vi "CFTS (TDT).vi"() -> ()   [LabVIEW 2020]
uses:
  Human Studies/NSDH Frontend/LV Source/Typedefs/NSDH-Options.ctl
  CFTS Main Panel SubVIs/CFTS-Experiment State.ctl
  <vilib>/Utility/sysdir.llb/System Directory Type.ctl
  DPOAE VIs/DP Analysis Panel.vi
  DPOAE VIs/DP I-O Main Panel.vi
  Calibration VIs/Calibrate Probe Tube.vi
panel:
  in  "Options":bool
  in  "CalMenu":u16(ring) items=["Calibration", "In-ear", "Probe tube", "Headphone"]
  out "exit signal":bool
  in  "DevicesButton":bool
  in  "DPAnalysisButton":bool
  in  "DPButton":bool
  in  "Cancel Button":bool
  in  "ApplyButton":bool
  in  "ID":string
  in  "Number":i32
  in  "EphysBrowserButton":bool
  in  "EphysButton":bool
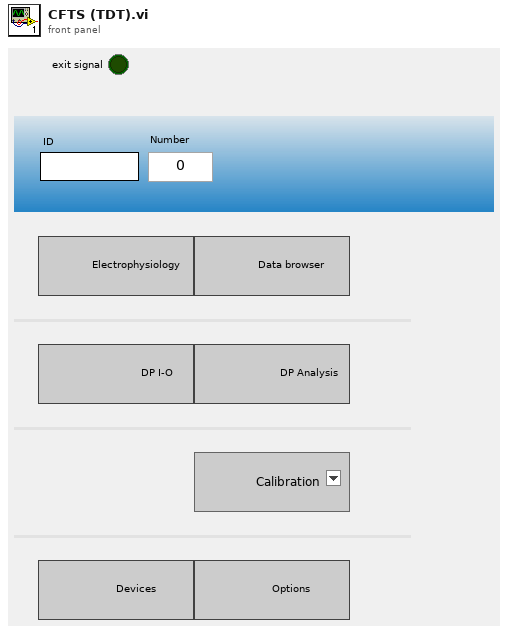
[diagram p1: front panel]
types:
  T1 = enum8{"Enabled", "Disabled", "Disabled and Grayed Out"}
  T2 = typedef "CFTS-Experiment State.ctl" = cluster{"Experimenter":string, "Number":u32, "Right":string, "Left":string, "Data Folder":path, "State File":path, "Version Info":string, "End Exposure Time":dbl, "Exposure Duration":string, "Run #":cluster{"CAP":i16, "ABR":i16, "DP":i16, "VsEP":i16, "MeasSeq":i16, "SubSeq":i16, "SFOAE":i16}}
  T3 = typedef "NSDH-Options.ctl" = cluster{"Data root":path}
  T4 = typedef "System Directory Type.ctl" = i32
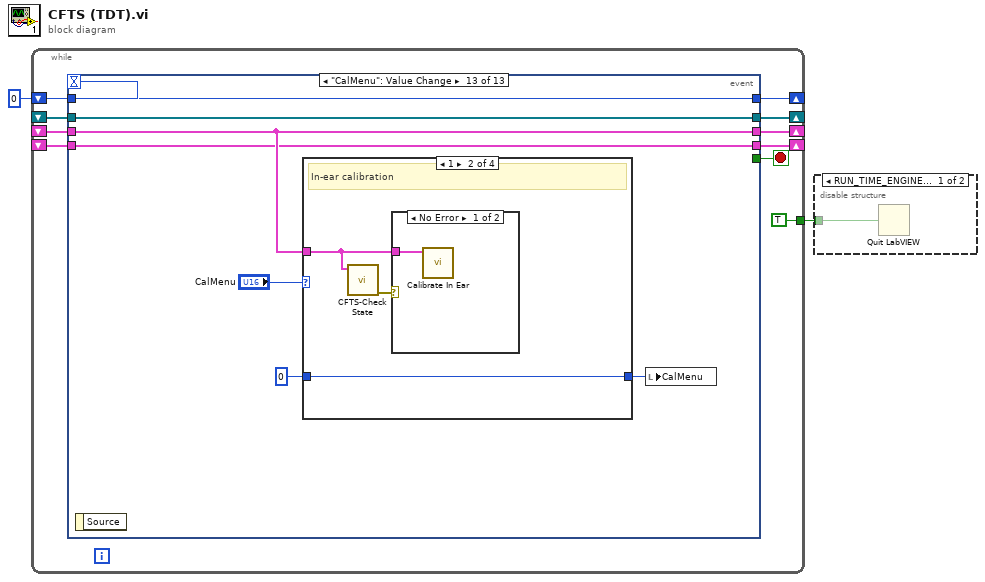
[diagram p0: block diagram]
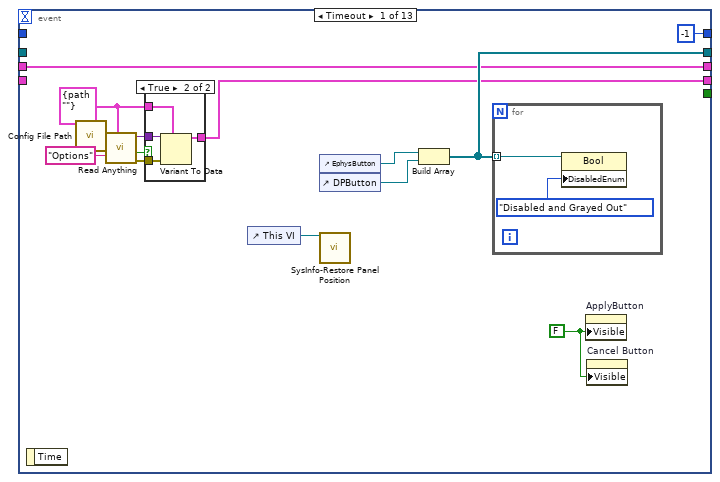
[diagram p3: hidden frame]
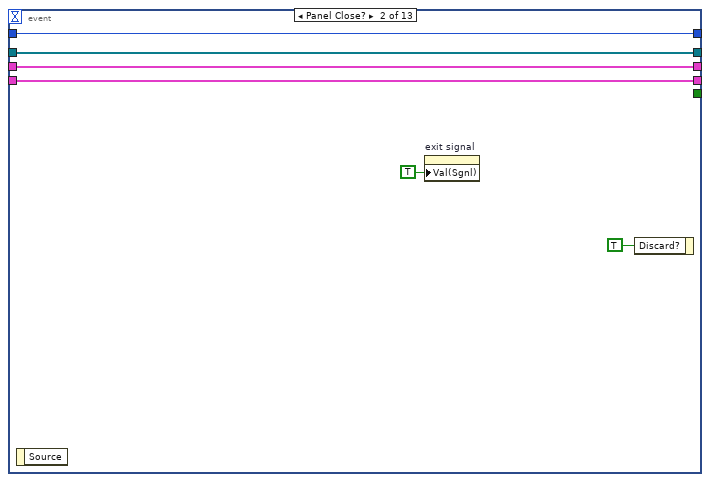
[diagram p5: hidden frame]
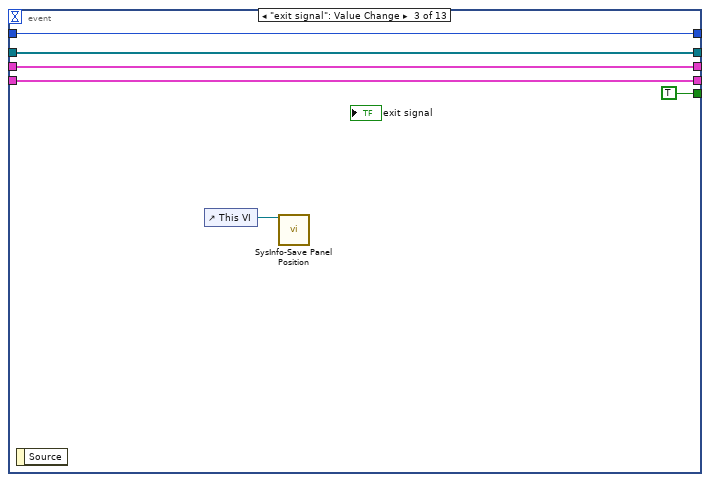
[diagram p6: hidden frame]
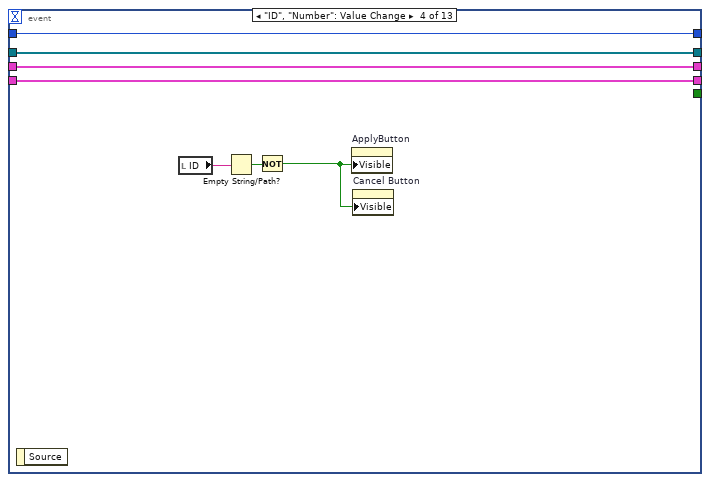
[diagram p7: hidden frame]
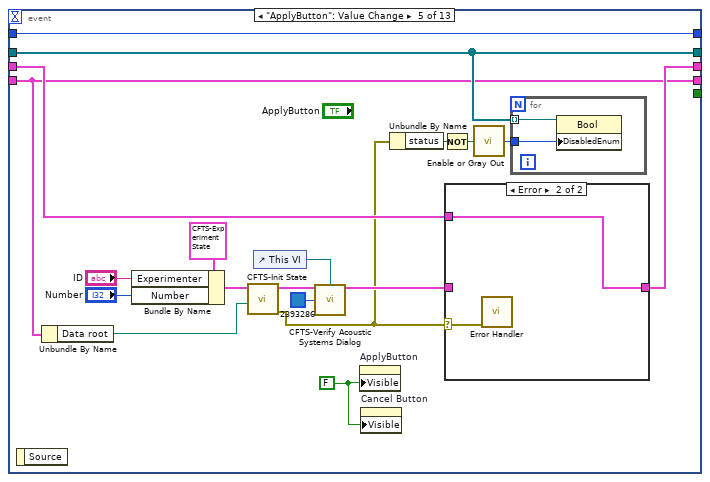
[diagram p8: hidden frame]
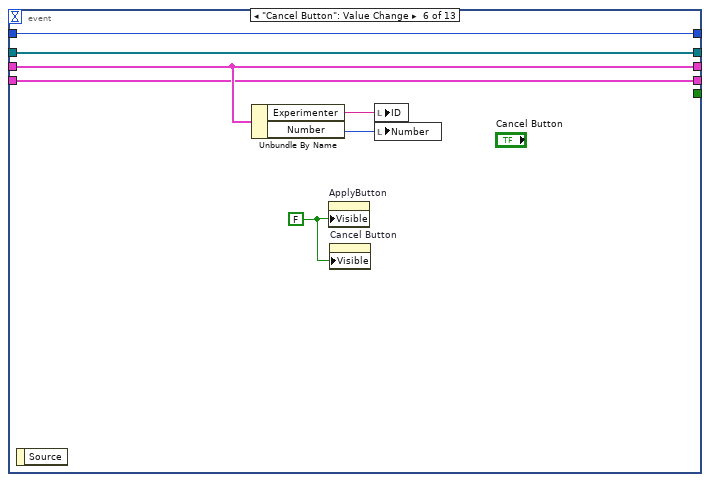
[diagram p10: hidden frame]
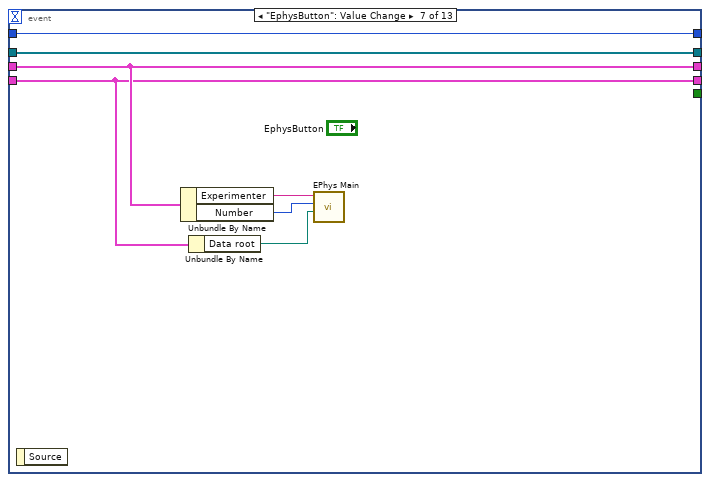
[diagram p11: hidden frame]
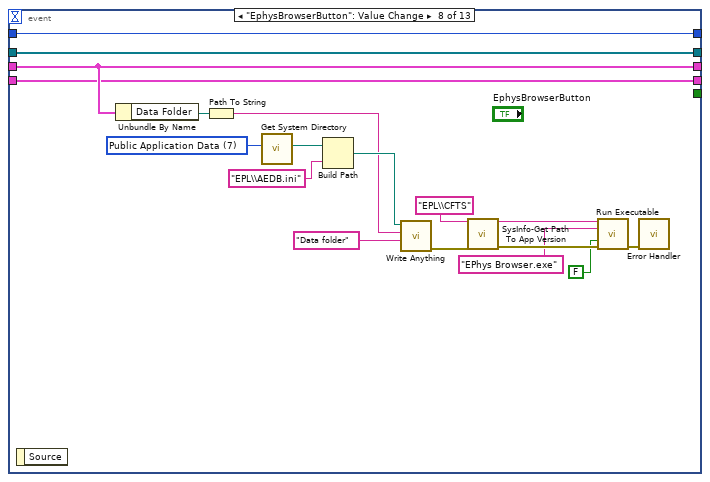
[diagram p12: hidden frame]
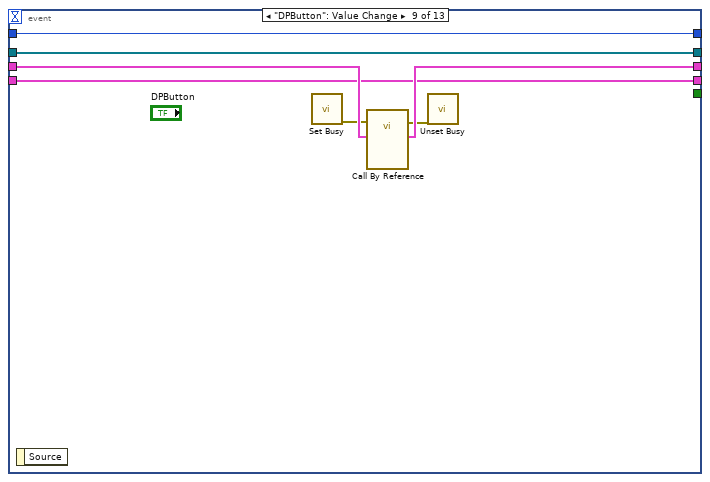
[diagram p13: hidden frame]
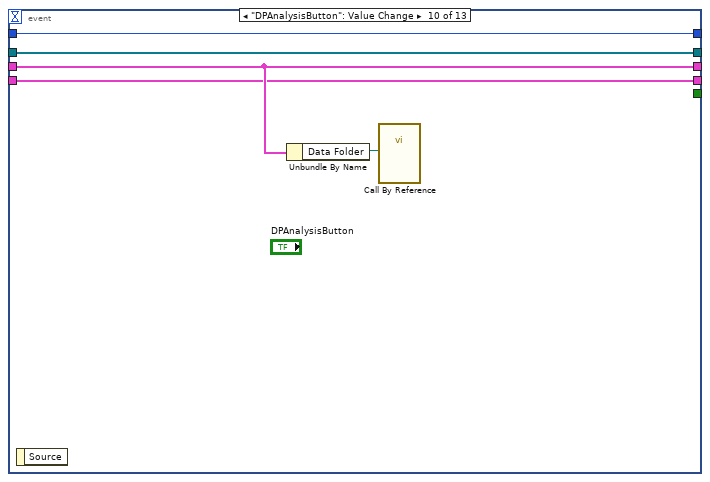
[diagram p14: hidden frame]
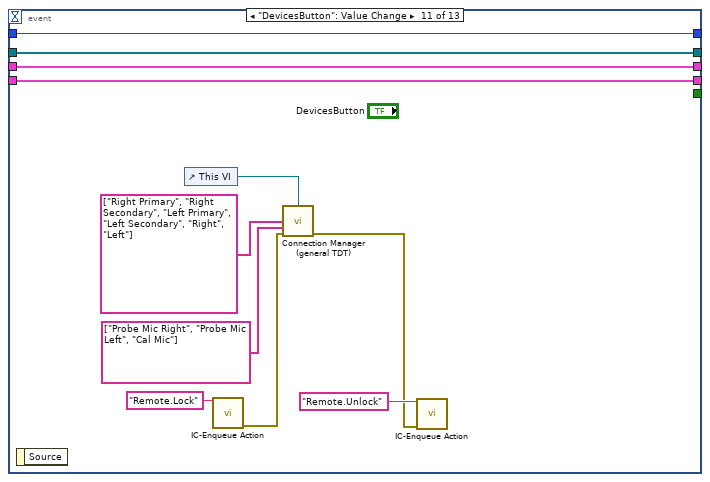
[diagram p15: hidden frame]
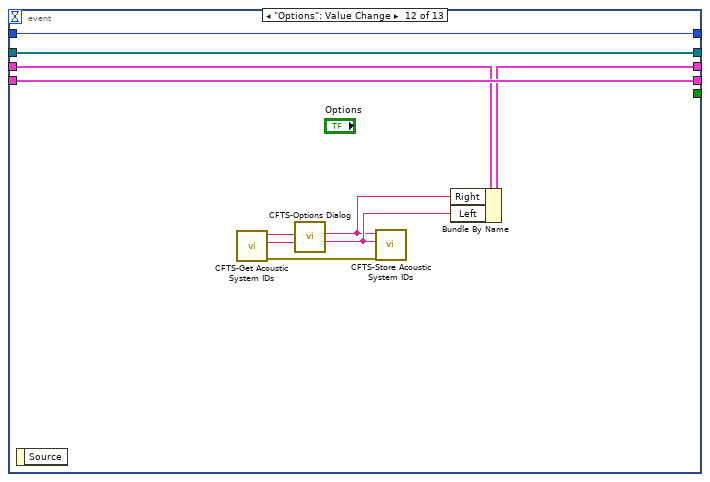
[diagram p16: hidden frame]
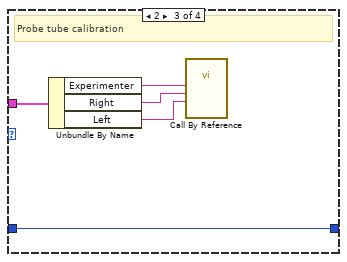
[diagram p19: hidden frame]
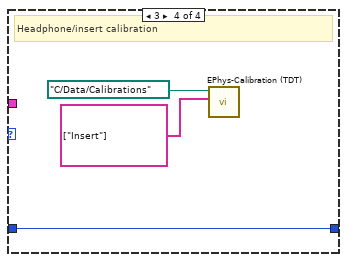
[diagram p20: hidden frame]
diagram:
  n1 = while {
    shift-right: [w11] -> _
    shift-left: 0 -> [w12]
    shift-right: [w9] -> _
    shift-left: _ -> [w8]
    shift-right: [w7] -> _
    shift-left: _ -> [w6]
    tunnel: [TRUE] -> w1
    shift-right: [w4] -> _
    shift-left: _ -> [w3]
    stop <- w10 stop-if-true
    n2 = event shown="[12] \"CalMenu\": Value Change" {
      selector: _ -> [_ _ _ _ _ _ _ _ _ _ _ _ _]
      dyn-events: _ -> [_ _ _ _ _ _ _ _ _ _ _ _ _]
      timeout: w12 -> [_ _ _ _ _ _ _ _ _ _ _ _ _]
      tunnel: w12 -> [_ w38 w45 w52 w71 w83 w90 w108 w115 w120 w131 w141 w148]
      tunnel: [-1 w38 w45 w52 w71 w83 w90 w108 w115 w120 w131 w141 w148] -> w11
      tunnel: [_ _ TRUE _ _ _ _ _ _ _ _ _ _] -> w10
      tunnel: [w23 w36 w42 w51 w64 w82 w89 w107 w114 w119 w130 w140 w147] -> w9
      tunnel: w8 -> [_ w36 w42 w51 w64 w82 w89 w107 w114 w119 w130 w140 w147]
      tunnel: [w20 w35 w41 w47 w66 w80 w88 w99 w112 w117 w129 w133 w145] -> w7
      tunnel: w6 -> [w20 w35 w41 w47 w65 w80 w88 w99 w113 w117 w129 w134 w145]
      tunnel: [w16 w34 w40 w46 w60 w77 w87 w91 w109 w116 w121 w135 w142] -> w4
      tunnel: w3 -> [_ w34 w40 w46 w60 w77 w87 w91 w109 w116 w121 w135 w142]
      event Timeout {
        w17 = T3 {"Data root"=path ""} ("Options")
        w22 = FALSE
        n3 = event-data() -> ()  [unwired: 1 in, 1 out]
        n4 = call "Config File Path.vi"() -> ("Default config file name"=w13:path)  [unwired: 1 in]
        n5 = call "Read Anything.vi"("Type of Anything"=w17, "Section Name (Name of \"Type of Anything\")"="Options" ("Section Name (Name of \"Type of Anything\")"), "Path (dialog)"=w13) -> ("Error Out"=w19:errorcluster, "Found?"=w15:bool, "Anything"=w18:variant)  [unwired: 6 in]
        n6 = case shown="True" w15 {
          tunnel: w19 -> [_ w31]
          tunnel: w18 -> [_ w30]
          tunnel: w17 -> [w27 w29]
          tunnel: [w27 w28] -> w16
          frame False {
          }
          frame True {
            n7 = Variant To Data(error in=w31, type=w29, Variant=w30) -> (data=w28:T3)  [unwired: 1 out]
          }
        }
        n8 = control-ref of="This VI"() -> (w21:refnum<vi>)
        n9 = control-ref of="EphysButton"() -> (w25:refnum<vi>)
        n10 = control-ref of="DPButton"() -> (w24:refnum<vi>)
        n11 = call "SysInfo-Restore Panel Position.vi"("VI Refnum"=w21) -> ()  [unwired: 12 in, 3 out]
        n12 = Build Array(w25, w24) -> (w23:refnum<vi>[])
        n13 = for {
          tunnel: w23 -> [w33] mode=indexing
          n14 = property class="Bool"(reference=w33, "DisabledEnum"=T1."Disabled and Grayed Out" ("Disabled")) -> ()  [unwired: 1 in, 2 out]
        }
        n15 = property on="ApplyButton" class="Bool"("Visible"=w22) -> ()  [unwired: 2 in, 2 out]
        n16 = property on="Cancel Button" class="Bool"("Visible"=w22) -> ()  [unwired: 2 in, 2 out]
      }
      event Panel Close? {
        n17 = event-data() -> ()  [unwired: 1 in, 1 out]
        n18 = property on="exit signal" class="Bool (strict)"("Val(Sgnl)"=TRUE ("Value (Signaling)")) -> ()  [unwired: 2 in, 2 out]
        n19 = event-data("Discard?"=TRUE) -> ()  [unwired: 1 in, 1 out]
      }
      event "exit signal": Value Change {
        n20 = event-data() -> ()  [unwired: 1 in, 1 out]
        n21 = control-ref of="This VI"() -> (w43:refnum<vi>)
        n22 = call "SysInfo-Save Panel Position.vi"("VI Refnum"=w43) -> ()  [unwired: 14 in, 1 out]
      }
      event "ID", "Number": Value Change {
        n23 = event-data() -> ()  [unwired: 1 in, 1 out]
        n24 = local read "ID"() -> (w50:string)
        n25 = Empty String/Path?(string/path=w50) -> (empty?=w49:bool)
        n26 = Not(x=w49) -> (.not. x?=w48:bool)
        n27 = property on="ApplyButton" class="Bool"("Visible"=w48) -> ()  [unwired: 2 in, 2 out]
        n28 = property on="Cancel Button" class="Bool"("Visible"=w48) -> ()  [unwired: 2 in, 2 out]
      }
      event "ApplyButton": Value Change {
        w62 = FALSE ("Visible")
        n29 = event-data() -> ()  [unwired: 1 in, 1 out]
        n30 = Unbundle By Name(w60) -> ("Data root"=w59:path)
        n31 = Bundle By Name(cluster=T2 {"Experimenter"="", "Number"=0, "Right"="", "Left"="", "Data Folder"=path "", "State File"=path "", "Version Info"="", "End Exposure Time"=0.0, "Exposure Duration"="", "Run #"={"CAP"=0, "ABR"=0, "DP"=0, "VsEP"=0, "MeasSeq"=0, "SubSeq"=0, "SFOAE"=0}} ("Expt State"), "Experimenter"="ID", "Number"="Number") -> (w67:T2)
        n32 = call "CFTS-Init State.vi"("Root folder"=w59, "Experiment State (in)"=w67) -> ("error out"=w54:errorcluster, "Experiment State (out)"=w57:T2)  [unwired: 8 in]
        n33 = control-ref of="This VI"() -> (w55:refnum<vi>)
        n34 = call "CFTS-Verify Acoustic Systems Dialog.vi"("Expt State"=w57, "center on"=w55, "color"=u32 2393286) -> ("Cluster out"=w56:T2)  [unwired: 11 in, 1 out]
        n35 = property on="ApplyButton" class="Bool"("Visible"=w62) -> ()  [unwired: 2 in, 2 out]
        n36 = property on="Cancel Button" class="Bool"("Visible"=w62) -> ()  [unwired: 2 in, 2 out]
        n37 = Unbundle By Name(w54) -> ("status"=w53:bool)
        n38 = Not(x=w53) -> (.not. x?=w61:bool)
        n39 = case shown="Error" w54 {
          selector: w54 -> [_ w76]
          tunnel: w56 -> [w74 _]
          tunnel: [w74 w75] -> w66
          tunnel: w65 -> [_ w75]
          frame No Error {
          }
          frame Error {
            n40 = call "Error Handler.vi"("error in (no error)"=w76) -> ()  [unwired: 13 in, 2 out]
          }
        }
        n41 = call "Enable or Gray Out.vi"("Boolean"=w61) -> ("Disabled"=w63:T1)
        n42 = for {
          tunnel: w64 -> [w73] mode=indexing
          tunnel: w63 -> [w72]
          n43 = property class="Bool"(reference=w73, "DisabledEnum"=w72) -> ()  [unwired: 1 in, 2 out]
        }
      }
      event "Cancel Button": Value Change {
        w81 = FALSE ("Visible")
        n44 = event-data() -> ()  [unwired: 1 in, 1 out]
        n45 = Unbundle By Name(w80) -> ("Experimenter"=w79:string, "Number"=w78:u32)
        n46 = property on="ApplyButton" class="Bool"("Visible"=w81) -> ()  [unwired: 2 in, 2 out]
        n47 = property on="Cancel Button" class="Bool"("Visible"=w81) -> ()  [unwired: 2 in, 2 out]
        n48 = local write "ID"(w79) -> ()
        n49 = local write "Number"(w78) -> ()
      }
      event "EphysButton": Value Change {
        n50 = event-data() -> ()  [unwired: 1 in, 1 out]
        n51 = Unbundle By Name(w88) -> ("Experimenter"=w86:string, "Number"=w85:u32)
        n52 = Unbundle By Name(w87) -> ("Data root"=w84:path)
        n53 = call "EPhys Main.vi"("root"=w84, "num"=w85, "id"=w86) -> ()  [unwired: 9 in]
      }
      event "EphysBrowserButton": Value Change {
        w95 = T4 7 items=["User Home", "User Desktop", "User Documents", "User Application Data", "User Preferences", "User Temporary", "Public Documents", "Public Application Data", "Public Preferences", "System Core Libraries", "System Installed Libraries", "Application Files", "Boot Volume Root"] ("system directory type")
        n54 = event-data() -> ()  [unwired: 1 in, 1 out]
        n55 = Unbundle By Name(w99) -> ("Data Folder"=w100:path)
        n56 = Path To String(path=w100) -> (string=w93:string)
        n57 = call <vilib>:"Get System Directory.vi"("system directory type"=w95) -> ("system directory"=w96:path)  [unwired: 10 in]
        n58 = Build Path(base path=w96, name or relative path="EPL\\AEDB.ini") -> (appended path=w94:path)
        n59 = call "Write Anything.vi"("Section Name (Name of \"Anything\")"="Data folder" ("Section Name (Name of \"Anything\")"), "Anything"=w93, "Path (dialog)"=w94) -> ("Error Out"=w98:errorcluster)  [unwired: 7 in, 1 out]
        n60 = call "SysInfo-Get Path To App Version.vi"("Path root"="EPL\\CFTS", "error in"=w98) -> ("Path with version"=w105:string, "error out"=w104:errorcluster)  [unwired: 11 in, 1 out]
        n61 = call "Run Executable.vi"("Folder"=w105, ".EXE name"="EPhys Browser.exe", "Wait (F)"=FALSE, "error in (no error)"=w104) -> ("error out"=w101:errorcluster)  [unwired: 11 in]
        n62 = call "Error Handler.vi"("error in (no error)"=w101) -> ()  [unwired: 13 in, 2 out]
      }
      event "DPButton": Value Change {
        n63 = event-data() -> ()  [unwired: 1 in, 1 out]
        n64 = call <vilib>:"Set Busy.vi"() -> ("error out"=w111:errorcluster)  [unwired: 10 in, 1 out]
        n65 = call-by-ref "?"(error in=w111, "Expt State (in)"=w113) -> (error out=w110:errorcluster, "State"=w112:T2)  [unwired: 11 in, 1 out]
        n66 = call <vilib>:"Unset Busy.vi"("error in (no error)"=w110) -> ()  [unwired: 10 in, 1 out]
      }
      event "DPAnalysisButton": Value Change {
        n67 = event-data() -> ()  [unwired: 1 in, 1 out]
        n68 = Unbundle By Name(w117) -> ("Data Folder"=w118:path)
        n69 = call-by-ref "?"("Data folder in"=w118) -> ()  [unwired: 13 in, 2 out]
      }
      event "DevicesButton": Value Change {
        n70 = event-data() -> ()  [unwired: 1 in, 1 out]
        n71 = control-ref of="This VI"() -> (w128:refnum<vi>)
        n72 = call "IC-Enqueue Action.vi"("Action"="Remote.Lock") -> ("error out"=w123:errorcluster)  [unwired: 14 in]
        n73 = call "Connection Manager (general TDT).vi"("Parent VI"=w128, "AO Endpoints"=string[] ["Right Primary", "Right Secondary", "Left Primary", "Left Secondary", "Right", "Left"], "AI Endpoints"=string[] ["Probe Mic Right", "Probe Mic Left", "Cal Mic"], "error in (no error)"=w123) -> ("error out"=w122:errorcluster)  [unwired: 8 in, 3 out]
        n74 = call "IC-Enqueue Action.vi"("Action"="Remote.Unlock", "error in (no error)"=w122) -> ()  [unwired: 13 in, 1 out]
      }
      event "Options": Value Change {
        n75 = event-data() -> ()  [unwired: 1 in, 1 out]
        n76 = call "CFTS-Get Acoustic System IDs.vi"() -> ("error out"=w139:errorcluster, "Left"=w137:string, "Right"=w138:string)  [unwired: 9 in]
        n77 = call "CFTS-Options Dialog.vi"("Left"=w137, "Right"=w138) -> ("Left out"=w136:string, "Right out"=w132:string)  [unwired: 7 in, 1 out]
        n78 = call "CFTS-Store Acoustic System IDs.vi"("error in (no error)"=w139, "Left"=w136, "Right"=w132) -> ()  [unwired: 8 in, 1 out]
        n79 = Bundle By Name(cluster=w134, "Right"=w132, "Left"=w136) -> (w133:T2)
      }
      event "CalMenu": Value Change {
        n80 = event-data() -> ()  [unwired: 1 in, 1 out]
        n81 = case shown="1" "CalMenu" {
          tunnel: w145 -> [_ w151 w154 _]
          tunnel: 0 -> [w149 w152 w158 w161]
          tunnel: [w149 w152 w158 w161] -> w143
          frame 0, Default {
          }
          frame 1 {
            # "In-ear calibration"
            n82 = call "CFTS-Check State.vi"("Expt State"=w151) -> ("error out"=w150:errorcluster)  [unwired: 10 in]
            n83 = case shown="No Error" w150 {
              tunnel: w151 -> [w153 _]
              frame No Error {
                n84 = call "Calibrate In Ear.vi"("State"=w153) -> ()  [unwired: 10 in, 1 out]
              }
              frame Error {
              }
            }
          }
          frame 2 {
            # "Probe tube calibration"
            n85 = Unbundle By Name(w154) -> ("Experimenter"=w157:string, "Right"=w155:string, "Left"=w156:string)
            n86 = call-by-ref "?"("Left"=w156, "Right"=w155, "User ID"=w157) -> ()  [unwired: 11 in, 2 out]
          }
          frame 3 {
            # "Headphone/insert calibration"
            n87 = call "EPhys-Calibration (TDT).vi"("Endpoints"=string[] ["Insert"], "Default Folder"=path "C:/Data/Calibrations") -> ()  [unwired: 10 in]
          }
        }
        n88 = local write "CalMenu"(w143) -> ()
      }
    }
  }
  n89 = disable-structure shown="RUN_TIME_ENGINE==True, Default" {
    disable-tunnel: w1 -> [w162 _]
    frame condition #0 {
      n90 = Quit LabVIEW(quit? (T)=w162) -> ()
    }
    frame condition #1 (active) {
    }
  }
